vi "FGV-BroadcastRegistry.vi"(0 "Source":string, 5 "Target":string, 7 "Status":string, 9 "API":string, 11 "Error In":errorcluster caption="error in (no error)", 12 "Operation":T1) -> (4 "Response Message":string[](array[string]), 15 "error out":errorcluster)   [LabVIEW 2017, in "Communicable State Machine.lvlib"]
doc: "### FGV-BroadcastRegistry.vi\n\n-- <b>Controls</b> --\n- <b>Source</b>:\n- <b>Target</b>:\n- <b>Status</b>:\n- <b>API</b>:\n- <b>Operation</b>:\n\n-- <b>Indicators</b> --\n- <b>response message</b>:"
uses:
  Communicable State Machine.lvlib
  Operation-BroadcastRegistry.ctl
  BroadcastRegistry/BroadcastRegistry.ctl
  ChangeFlag/ChangeFlag-Write.vi
  Utility/Random Change Flag.vi
  ChangeFlag/ChangeFlagDB.vi
  _Shared/CSM Shared.lvlib
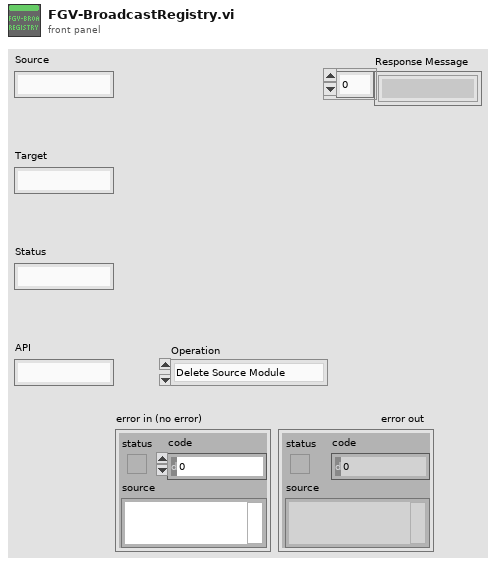
[diagram p1: front panel]
types:
  T1 = typedef "Communicable State Machine.lvlib/Operation-BroadcastRegistry.ctl" = enum16{"Delete Source Module", "Delete Target Module", "Remove Module", "Register", "Unregister", "Check", "List Status", "List Entries", "List Status Of Source", "Drop"}
  T2 = typedef "Communicable State Machine.lvlib/BroadcastRegistry.ctl" = cluster{"RegistryTable":variant}
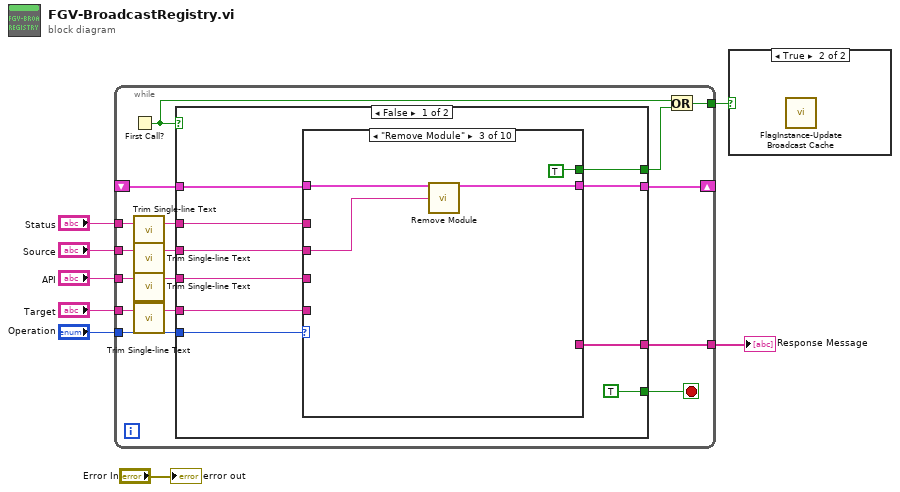
[diagram p0: block diagram]
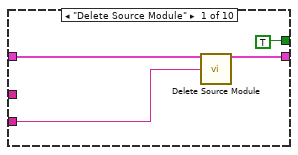
[diagram p2: hidden frame]
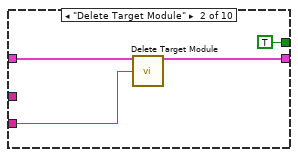
[diagram p3: hidden frame]
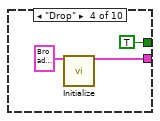
[diagram p4: hidden frame]
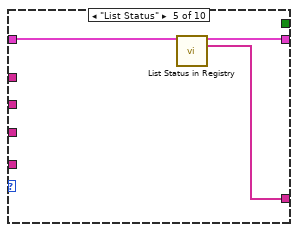
[diagram p5: hidden frame]
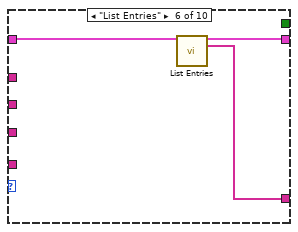
[diagram p6: hidden frame]
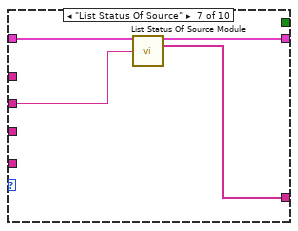
[diagram p7: hidden frame]
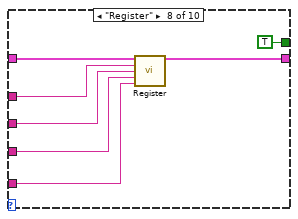
[diagram p8: hidden frame]
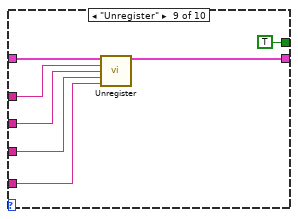
[diagram p9: hidden frame]
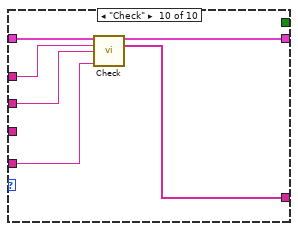
[diagram p10: hidden frame]
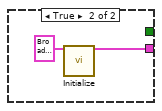
[diagram p11: hidden frame]
diagram:
  n1 = while {
    shift-right: [w23] -> _
    shift-left: _ -> [w22]
    tunnel: "Operation" -> [w21]
    tunnel: "Target" -> [w14]
    tunnel: "Source" -> [w13]
    tunnel: "Status" -> [w15]
    tunnel: "API" -> [w16]
    tunnel: [w20] -> w3
    tunnel: [w17] -> w1
    stop <- w24 stop-if-true
    n2 = First Call?() -> (First Call?: T/F=w18:bool)
    n3 = call "Trim Single-line Text.vi"("single-line text"=w15) -> ("trimed text"=w10:string)  [unwired: 2 in]
    n4 = call "Trim Single-line Text.vi"("single-line text"=w13) -> ("trimed text"=w12:string)  [unwired: 2 in]
    n5 = call "Trim Single-line Text.vi"("single-line text"=w16) -> ("trimed text"=w9:string)  [unwired: 2 in]
    n6 = call "Trim Single-line Text.vi"("single-line text"=w14) -> ("trimed text"=w11:string)  [unwired: 2 in]
    n7 = case shown="False" w18 {
      tunnel: [TRUE _] -> w24
      tunnel: [w25 w81] -> w23
      tunnel: w22 -> [w26 _]
      tunnel: w21 -> [w33 _]
      tunnel: w11 -> [w32 _]
      tunnel: w12 -> [w31 _]
      tunnel: w10 -> [w30 _]
      tunnel: w9 -> [w29 _]
      tunnel: [w28 _] -> w20
      tunnel: [w27 _] -> w19
      frame False {
        n8 = case shown="\"Remove Module\"" w33 {
          tunnel: [w36 w40 w44 w47 w51 w54 w58 w65 w71 w78] -> w25
          tunnel: w26 -> [w37 w41 w45 _ w52 w55 w59 w64 w72 w79]
          tunnel: w32 -> [_ _ _ _ _ _ _ w60 w68 w76]
          tunnel: w31 -> [w35 w39 w43 _ _ _ w57 w62 w69 w75]
          tunnel: w30 -> [_ _ _ _ _ _ _ w63 w70 w74]
          tunnel: w29 -> [_ _ _ _ _ _ _ w61 w67 _]
          tunnel: [_ _ _ _ w50 w53 w56 _ _ w77] -> w28
          tunnel: [TRUE ("Cache changed?") TRUE ("Cache changed?") TRUE ("Cache changed?") TRUE ("Cache changed?") _ _ _ TRUE ("Cache changed?") TRUE ("Cache changed?") _] -> w27
          frame "Delete Source Module" {
            n9 = call "Delete Source Module.vi"("BroadcastRegistry In"=w37, "Source"=w35) -> ("BroadcastRegistry Out"=w36:T2)  [unwired: 13 in]
          }
          frame "Delete Target Module" {
            n10 = call "Delete Target Module.vi"("BroadcastRegistry In"=w41, "Source"=w39) -> ("BroadcastRegistry Out"=w40:T2)  [unwired: 13 in]
          }
          frame "Remove Module" {
            n11 = call "Remove Module.vi"("BroadcastRegistry In"=w45, "Source"=w43) -> ("BroadcastRegistry Out"=w44:T2)  [unwired: 13 in]
          }
          frame "Drop" {
            n12 = call "Initialize.vi"("BroadcastRegistry In"=T2 {"RegistryTable"=variant}) -> ("BroadcastRegistry Out"=w47:T2)  [unwired: 14 in]
          }
          frame "List Status" {
            n13 = call "List Status in Registry.vi"("BroadcastRegistry In"=w52) -> ("BroadcastRegistry Out"=w51:T2, "Status"=w50:string[])  [unwired: 13 in]
          }
          frame "List Entries" {
            n14 = call "List Entries.vi"("BroadcastRegistry In"=w55) -> ("BroadcastRegistry Out"=w54:T2, "Array"=w53:string[])  [unwired: 13 in]
          }
          frame "List Status Of Source" {
            n15 = call "List Status Of Source Module.vi"("BroadcastRegistry In"=w59, "Source"=w57) -> ("BroadcastRegistry Out"=w58:T2, "Array"=w56:string[])  [unwired: 12 in]
          }
          frame "Register" {
            n16 = call "Register.vi"("BroadcastRegistry In"=w64, "Status"=w63, "Source"=w62, "Api"=w61, "Target"=w60) -> ("BroadcastRegistry Out"=w65:T2)  [unwired: 10 in]
          }
          frame "Unregister" {
            n17 = call "Unregister.vi"("BroadcastRegistry In"=w72, "Status"=w70, "Source"=w69, "Api"=w67, "Target"=w68) -> ("BroadcastRegistry Out"=w71:T2)  [unwired: 10 in]
          }
          frame "Check" {
            n18 = call "Check.vi"("BroadcastRegistry In"=w79, "Status"=w74, "Source"=w75, "Target"=w76) -> ("BroadcastRegistry Out"=w78:T2, "Response Message Info"=w77:string[])  [unwired: 10 in]
          }
        }
      }
      frame True {
        n19 = call "Initialize.vi"("BroadcastRegistry In"=T2 {"RegistryTable"=variant}) -> ("BroadcastRegistry Out"=w81:T2)  [unwired: 14 in]
      }
    }
    n20 = Or(x=w18, y=w19) -> (x .or. y?=w17:bool)
  }
  "Response Message" <- w3
  n21 = case shown="True" w1 {
    frame False {
    }
    frame True {
      n22 = call "FlagInstance-Update Broadcast Cache.vi"() -> ()  [unwired: 10 in, 2 out]
    }
  }
  "error out" <- "Error In"
